vi "AssemblyArea.vi"(4 "Current Hopper Val":bool, 6 "Prev Hopper Val":bool, 8 "Program Control":bool, 9 "Hopper Detect":bool, 10 "Pegs":refnum<vi>, 11 "RingQ":refnum<vi>) -> (3 "Hopper Solenoid":bool)   [LabVIEW 2016]
panel:
  in  "Algorithm: Catch Some (T) / Catch All (F)":bool
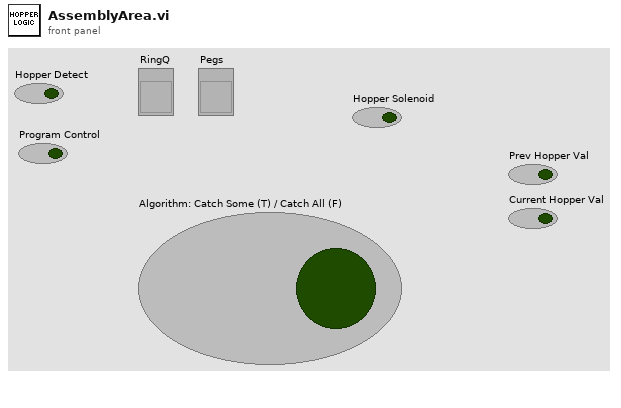
[diagram p1: front panel]
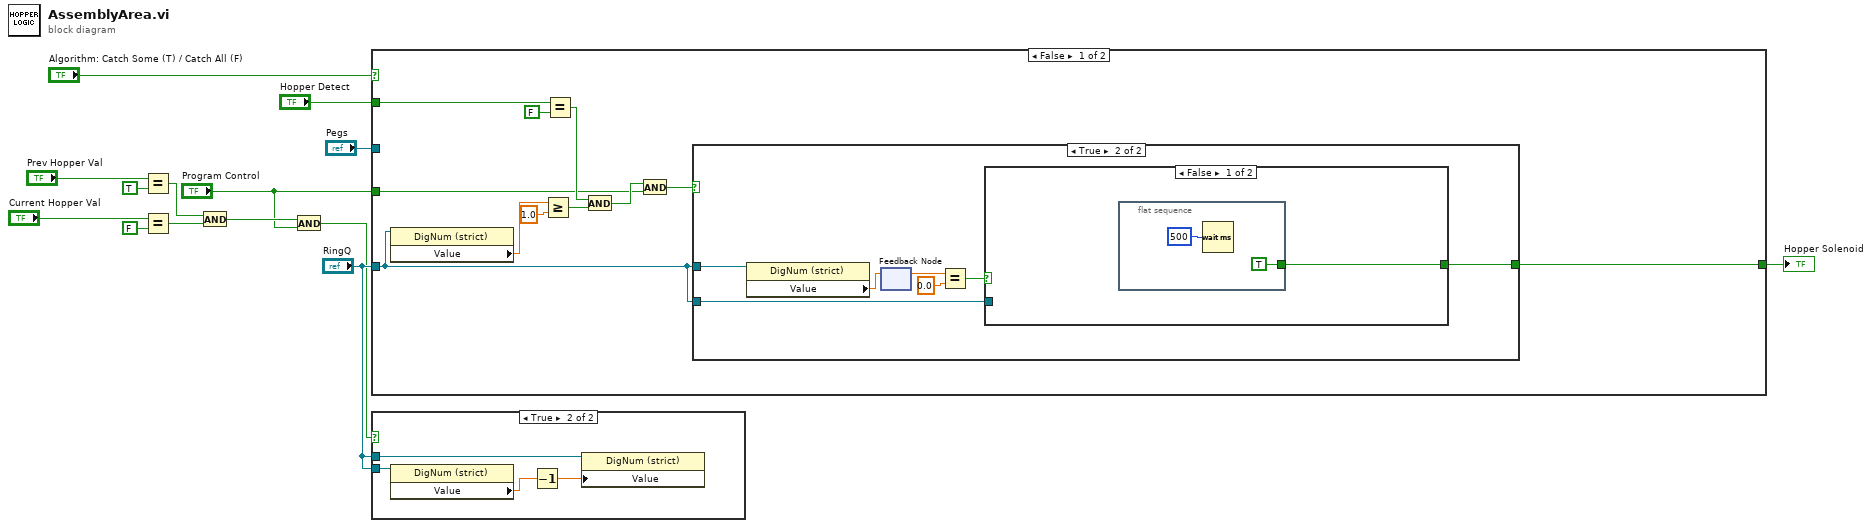
[diagram p0: block diagram]
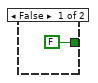
[diagram p3: hidden frame]
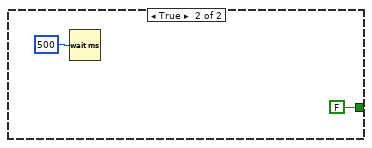
[diagram p4: hidden frame]
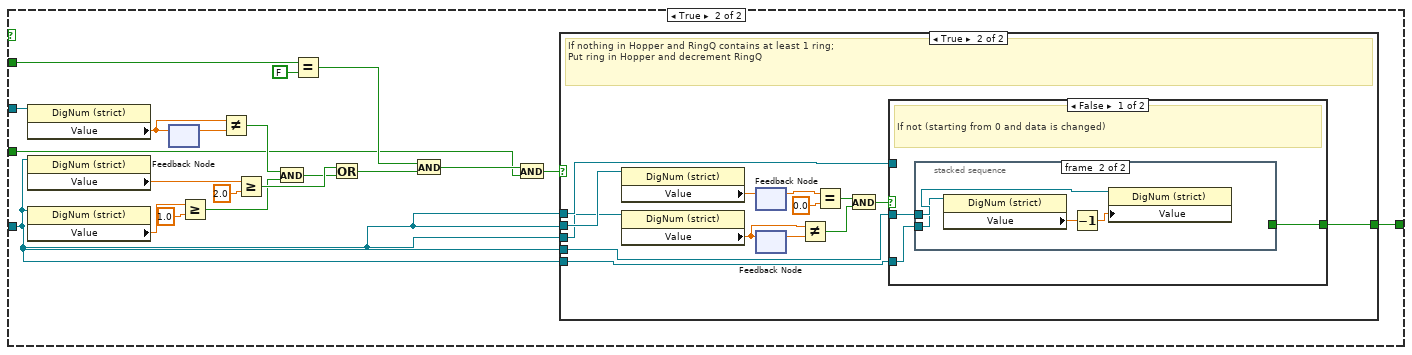
[diagram p5: hidden frame]
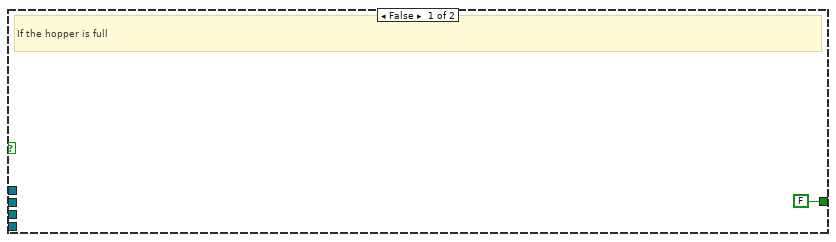
[diagram p6: hidden frame]
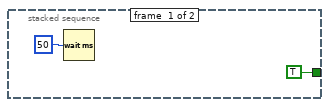
[diagram p7: hidden frame]
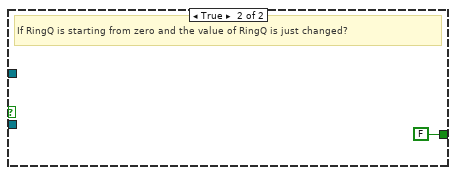
[diagram p8: hidden frame]
diagram:
  n1 = Equal?(x="Prev Hopper Val", y=TRUE) -> (x = y?=w9:bool)
  n2 = Equal?(x="Current Hopper Val", y=FALSE) -> (x = y?=w10:bool)
  n3 = And(x=w9, y=w10) -> (x .and. y?=w3:bool)
  n4 = And(x=w3, y="Program Control") -> (x .and. y?=w1:bool)
  n5 = case shown="False" "Algorithm: Catch Some (T) / Catch All (F)" {
    tunnel: [w19 w56] -> w14
    tunnel: "Hopper Detect" -> [w25 w54]
    tunnel: "RingQ" -> [w16 w41]
    tunnel: "Pegs" -> [_ w40]
    tunnel: "Program Control" -> [w15 w39]
    frame False {
      n6 = property class="DigNum (strict)"(reference=w16) -> ("Value"=w22:dbl)  [unwired: 1 in, 2 out]
      n7 = Greater Or Equal?(x=w22, y=1.0) -> (x >= y?=w20:bool)
      n8 = Equal?(x=w25, y=FALSE) -> (x = y?=w23:bool)
      n9 = And(x=w23, y=w20) -> (x .and. y?=w18:bool)
      n10 = And(x=w18, y=w15) -> (x .and. y?=w17:bool)
      n11 = case shown="True" w17 {
        tunnel: [FALSE w29] -> w19
        tunnel: w16 -> [_ w28]
        tunnel: w16 -> [_ w27]
        frame False {
        }
        frame True {
          n12 = property class="DigNum (strict)"(reference=w28) -> ("Value"=w33:dbl)  [unwired: 1 in, 2 out]
          n13 = feedback #1() -> (w32:dbl)  [unwired: 1 in]
          n14 = feedback-in #1(w33) -> ()
          n15 = Equal?(x=w32, y=0.0) -> (x = y?=w30:bool)
          n16 = case shown="False" w30 {
            tunnel: [w34 FALSE] -> w29
            tunnel: w27 -> [_ _]
            frame False {
              n17 = flat-sequence {
                tunnel: [TRUE] -> w34
                frame #0 {
                  n18 = Wait (ms)(milliseconds to wait=u32 500) -> ()  [unwired: 1 out]
                }
              }
            }
            frame True {
              n19 = Wait (ms)(milliseconds to wait=u32 500) -> ()  [unwired: 1 out]
            }
          }
        }
      }
    }
    frame True {
      n20 = property class="DigNum (strict)"(reference=w40) -> ("Value"=w57:dbl)  [unwired: 1 in, 2 out]
      n21 = property class="DigNum (strict)"(reference=w41) -> ("Value"=w47:dbl)  [unwired: 1 in, 2 out]
      n22 = property class="DigNum (strict)"(reference=w41) -> ("Value"=w46:dbl)  [unwired: 1 in, 2 out]
      n23 = feedback #2() -> (w58:dbl)  [unwired: 1 in]
      n24 = feedback-in #2(w57) -> ()
      n25 = Greater Or Equal?(x=w46, y=1.0) -> (x >= y?=w50:bool)
      n26 = Not Equal?(x=w57, y=w58) -> (x != y?=w45:bool)
      n27 = Greater Or Equal?(x=w47, y=2.0) -> (x >= y?=w52:bool)
      n28 = And(x=w45, y=w50) -> (x .and. y?=w48:bool)
      n29 = Equal?(x=w54, y=FALSE) -> (x = y?=w43:bool)
      n30 = Or(x=w52, y=w48) -> (x .or. y?=w44:bool)
      n31 = And(x=w43, y=w44) -> (x .and. y?=w42:bool)
      n32 = And(x=w42, y=w39) -> (x .and. y?=w53:bool)
      n33 = case shown="True" w53 {
        tunnel: [FALSE w70] -> w56
        tunnel: w41 -> [_ w69]
        tunnel: w41 -> [_ w68]
        tunnel: w41 -> [_ w67]
        tunnel: w41 -> [_ w66]
        tunnel: w41 -> [_ w63]
        frame False {
          # "If the hopper is full"
        }
        frame True {
          # "If nothing in Hopper and RingQ contains at least 1 ring;\nPut ring in Hopper and decrement RingQ"
          n34 = property class="DigNum (strict)"(reference=w69) -> ("Value"=w73:dbl)  [unwired: 1 in, 2 out]
          n35 = property class="DigNum (strict)"(reference=w63) -> ("Value"=w65:dbl)  [unwired: 1 in, 2 out]
          n36 = feedback #3() -> (w72:dbl)  [unwired: 1 in]
          n37 = feedback-in #3(w73) -> ()
          n38 = feedback #4() -> (w64:dbl)  [unwired: 1 in]
          n39 = feedback-in #4(w65) -> ()
          n40 = Not Equal?(x=w65, y=w64) -> (x != y?=w62:bool)
          n41 = Equal?(x=w72, y=0.0) -> (x = y?=w61:bool)
          n42 = And(x=w61, y=w62) -> (x .and. y?=w60:bool)
          n43 = case shown="False" w60 {
            tunnel: [w76 FALSE] -> w70
            tunnel: w68 -> [w74 _]
            tunnel: w67 -> [w75 _]
            tunnel: w66 -> [_ _]
            frame False {
              # "If not (starting from 0 and data is changed)"
              n44 = stacked-sequence {
                tunnel: w75 -> [_ w80]
                tunnel: w74 -> [_ w79]
                tunnel: [TRUE _] -> w76
                frame #0 {
                  n45 = Wait (ms)(milliseconds to wait=u32 50) -> ()  [unwired: 1 out]
                }
                frame #1 {
                  n46 = property class="DigNum (strict)"(reference=w79) -> ("Value"=w82:dbl)  [unwired: 1 in, 2 out]
                  n47 = Decrement(x=w82) -> (x-1=w81:dbl)
                  n48 = property class="DigNum (strict)"(reference=w80, "Value"=w81) -> ()  [unwired: 1 in, 2 out]
                }
              }
            }
            frame True {
              # "If RingQ is starting from zero and the value of RingQ is just changed?"
            }
          }
        }
      }
    }
  }
  "Hopper Solenoid" <- w14
  n49 = case shown="True" w1 {
    tunnel: "RingQ" -> [_ w85]
    tunnel: "RingQ" -> [_ w84]
    frame False {
    }
    frame True {
      n50 = property class="DigNum (strict)"(reference=w85) -> ("Value"=w86:dbl)  [unwired: 1 in, 2 out]
      n51 = Decrement(x=w86) -> (x-1=w87:dbl)
      n52 = property class="DigNum (strict)"(reference=w84, "Value"=w87) -> ()  [unwired: 1 in, 2 out]
    }
  }
